vi "Sub_Initialization.vi"() -> (0 "SerialNumber":string, 1 "DeviceHandle":u32, 2 "TotalDevices":u32)   [LabVIEW 2013]
uses:
  x64_lib/Mightex_LEDDriver_SDK.dll
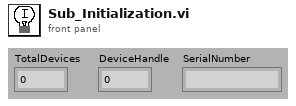
[diagram p1: front panel]
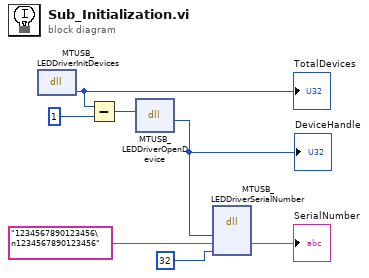
[diagram p0: block diagram]
diagram:
  n1 = dll-call lib="C:/Users/ignacio/Desktop/Patrick's File Reader Function/led_control/documentation/SDK/x64_lib/Mightex_LEDDriver_SDK.dll" fn="MTUSB_LEDDriverInitDevices"() -> ("return type"=w6:u32)  [unwired: 3 in, 2 out]
  "TotalDevices" <- w6
  n2 = Subtract(x=w6, y=1) -> (x-y=w5:u32)
  n3 = dll-call lib="C:/Users/ignacio/Desktop/Patrick's File Reader Function/led_control/documentation/SDK/x64_lib/Mightex_LEDDriver_SDK.dll" fn="MTUSB_LEDDriverOpenDevice"("arg1"=w5) -> ("return type"=w2:u32)  [unwired: 4 in, 2 out]
  "DeviceHandle" <- w2
  n4 = dll-call lib="C:/Users/ignacio/Desktop/Patrick's File Reader Function/led_control/documentation/SDK/x64_lib/Mightex_LEDDriver_SDK.dll" fn="MTUSB_LEDDriverSerialNumber"("arg1"=w2, "arg2"="1234567890123456\n1234567890123456", "arg3"=u32 32) -> ("arg2"=→"SerialNumber":string)  [unwired: 6 in, 2 out]
